vi "DeleteDuplicates.vi"(8 "error in (no error)":errorcluster, 11 "Array in":string[][](array[string])) -> (0 "error out":errorcluster, 3 "Array out":string[][](array[string]))   [LabVIEW 2015]
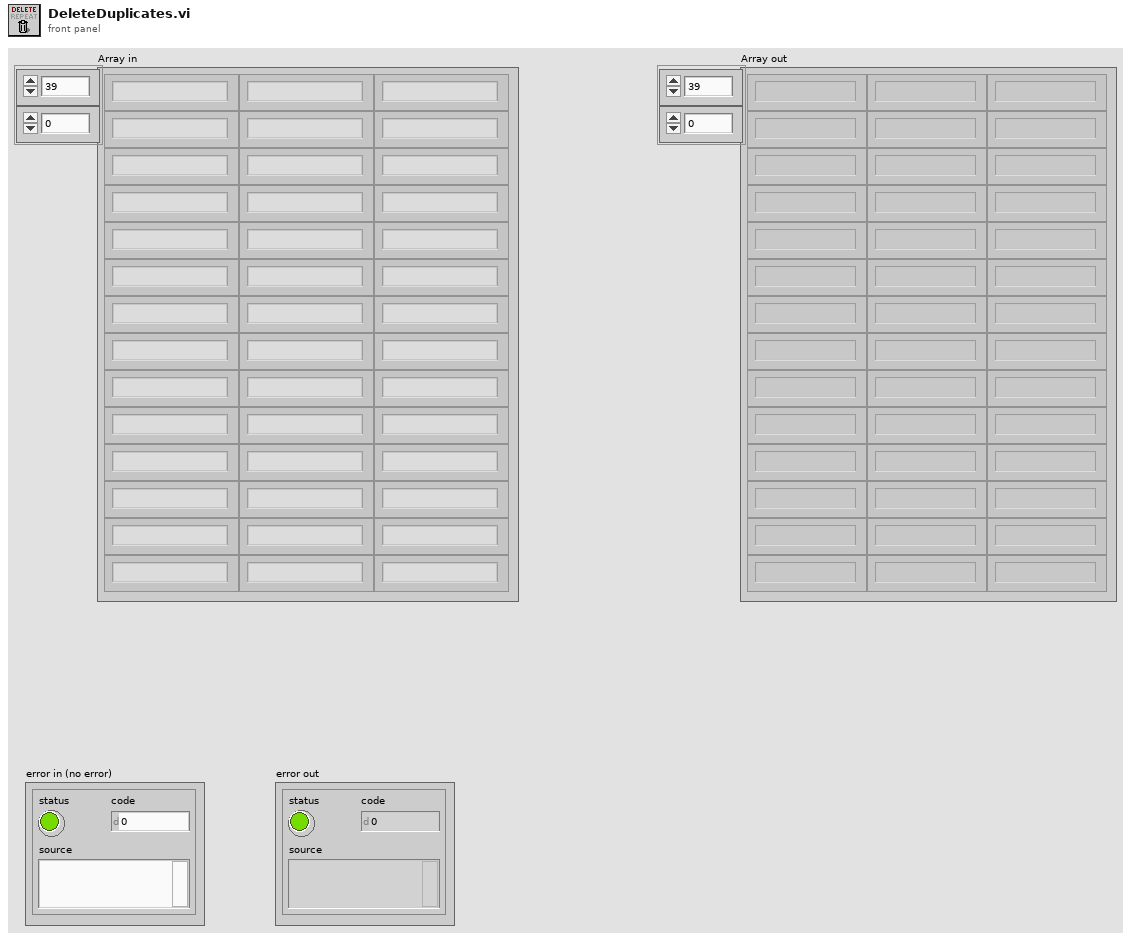
[diagram p1: front panel]
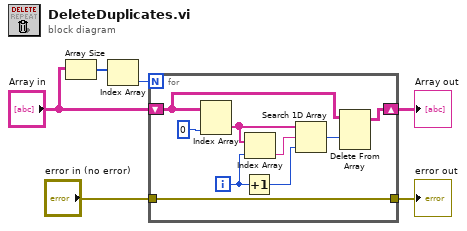
[diagram p0: block diagram]
diagram:
  n1 = Array Size(array="Array in") -> (size(s)=w6:i32[])
  n2 = Index Array(array=w6) -> (element=w5:i32)  [unwired: 1 in]
  n3 = for {
    N: w5 -> [_]
    shift-right: [w8] -> w3
    shift-left: "Array in" -> [w13]
    tunnel: [w7] -> w2
    tunnel: "error in (no error)" -> [w7]
    i -> [w10]
    n4 = Index Array(array=w13, index (col)=0) -> (element=w11:string[])  [unwired: 1 in]
    n5 = Increment(x=w10) -> (x+1=w12:i32)
    n6 = Index Array(array=w11, index=w10) -> (element=w9:string)
    n7 = Search 1D Array(1D array=w11, element=w9, start index (0)=w12) -> (index of element=w14:i32)
    n8 = Delete From Array(array=w13, index (row)=w14) -> (array with subset deleted=w8:string[][])  [unwired: 2 in, 1 out]
  }
  "Array out" <- w3
  "error out" <- w2
